vi "johnson.vi"() -> ()   [LabVIEW 2025]
uses:
  <vilib>/Analysis/1siggen.llb/Ramp Pattern by Samples.vi
  <vilib>/Analysis/NI_AALBase.lvlib
panel:
  out "Variance":dbl
  out "Stdev":dbl
  out "Mean":dbl
  out "Waveform Graph":dbl[][](graph)
  out "Output":string
  out "XY Graph":cluster{"Y":dbl[], "Y":dbl[]}[](graph)
  in  "samples":dbl
  in  "V/div":dbl
  in  "s/div":dbl
  in  "VISA resource name":refnum<visa-resource-name>
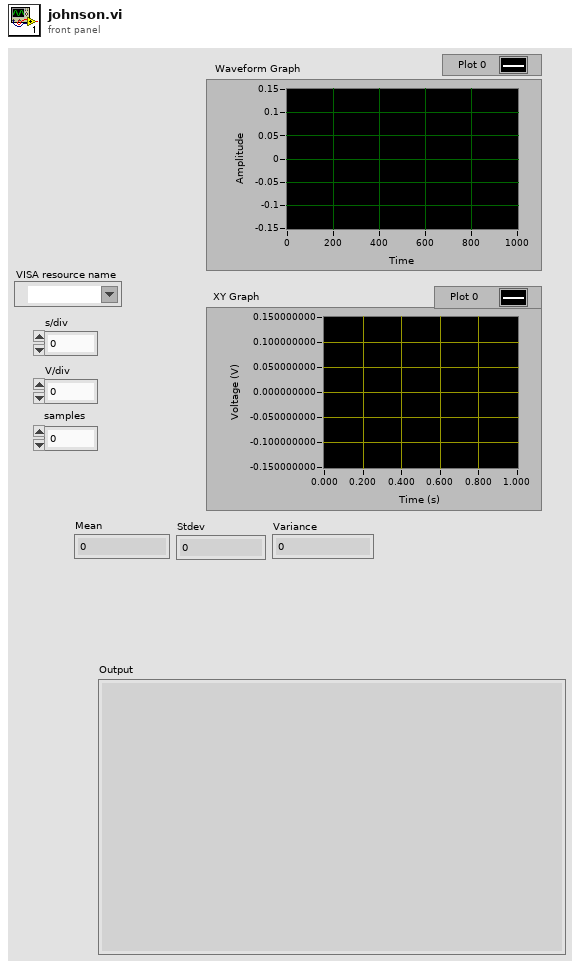
[diagram p1: front panel]
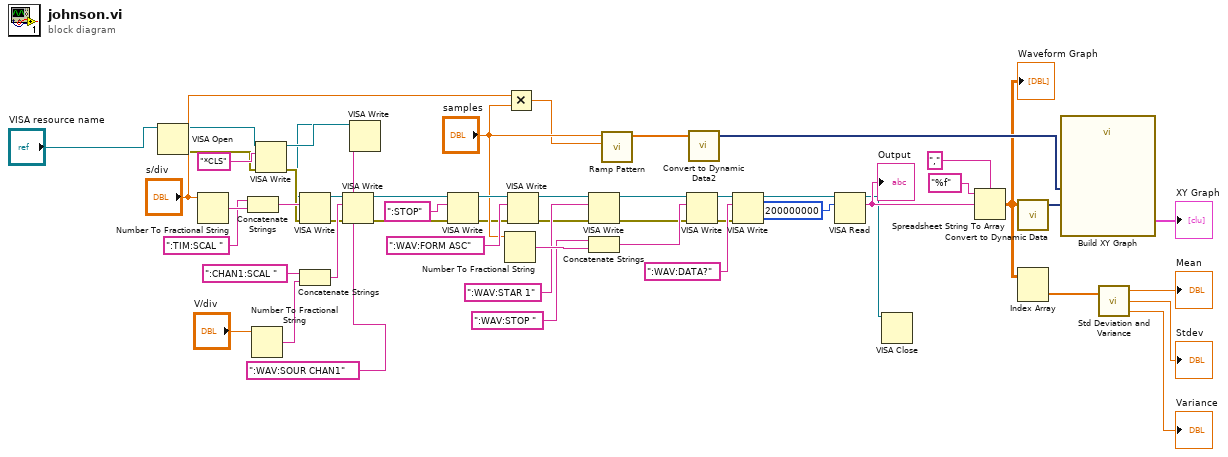
[diagram p0: block diagram]
diagram:
  n1 = VISA Open(VISA resource name="VISA resource name") -> (VISA resource name=w14:refnum<visa-resource-name>, error out=w11:errorcluster)  [unwired: 4 in]
  n2 = Number To Fractional String(number="s/div") -> (F-format string=w52:string)  [unwired: 3 in]
  n3 = Concatenate Strings(":TIM:SCAL ", w52) -> (w50:string)
  n4 = Number To Fractional String(number="V/div") -> (F-format string=w48:string)  [unwired: 3 in]
  n5 = VISA Write(VISA resource name=w14, write buffer="*CLS", error in (no error)=w11) -> (VISA resource name out=w2:refnum<visa-resource-name>, error out=w10:errorcluster)  [unwired: 1 out]
  n6 = Concatenate Strings(":CHAN1:SCAL ", w48) -> (w45:string)
  n7 = VISA Write(VISA resource name=w2, write buffer=":WAV:SOUR CHAN1") -> (VISA resource name out=w1:refnum<visa-resource-name>)  [unwired: 1 in, 2 out]
  n8 = VISA Write(VISA resource name=w1, write buffer=w50, error in (no error)=w10) -> (VISA resource name out=w46:refnum<visa-resource-name>, error out=w9:errorcluster)  [unwired: 1 out]
  n9 = VISA Write(VISA resource name=w46, write buffer=w45, error in (no error)=w9) -> (VISA resource name out=w43:refnum<visa-resource-name>, error out=w8:errorcluster)  [unwired: 1 out]
  n10 = VISA Write(VISA resource name=w43, write buffer=":STOP", error in (no error)=w8) -> (VISA resource name out=w33:refnum<visa-resource-name>, error out=w7:errorcluster)  [unwired: 1 out]
  n11 = Number To Fractional String(number="samples") -> (F-format string=w42:string)  [unwired: 3 in]
  n12 = Multiply(x="s/div", y="samples") -> (x*y=w21:dbl)
  n13 = VISA Write(VISA resource name=w33, write buffer=":WAV:FORM ASC", error in (no error)=w7) -> (VISA resource name out=w31:refnum<visa-resource-name>, error out=w6:errorcluster)  [unwired: 1 out]
  n14 = VISA Write(VISA resource name=w31, write buffer=":WAV:STAR 1", error in (no error)=w6) -> (VISA resource name out=w34:refnum<visa-resource-name>, error out=w5:errorcluster)  [unwired: 1 out]
  n15 = Concatenate Strings(":WAV:STOP ", w42) -> (w40:string)
  n16 = call-poly <vilib>:"Ramp Pattern.vi"("end"=w21, "samples"="samples") -> ("Ramp Pattern"=w28:dbl[])  [unwired: 8 in, 1 out]
  n17 = VISA Write(VISA resource name=w34, write buffer=w40, error in (no error)=w5) -> (VISA resource name out=w38:refnum<visa-resource-name>, error out=w4:errorcluster)  [unwired: 1 out]
  n18 = call "Convert to Dynamic Data2"("Array"=w28) -> ("Dynamic Data Type"=w26:dynamicdata)  [unwired: 3 in]
  n19 = VISA Write(VISA resource name=w38, write buffer=":WAV:DATA?", error in (no error)=w4) -> (VISA resource name out=w37:refnum<visa-resource-name>)  [unwired: 2 out]
  n20 = VISA Read(VISA resource name=w37, byte count=u32 200000000) -> (VISA resource name out=w12:refnum<visa-resource-name>, read buffer=w27:string)  [unwired: 1 in, 2 out]
  "Output" <- w27
  n21 = VISA Close(VISA resource name=w12) -> ()  [unwired: 1 in, 1 out]
  n22 = Spreadsheet String To Array(delimiter (Tab)=",", format string="%f", spreadsheet string=w27) -> (array=w20:dbl[][])  [unwired: 1 in]
  "Waveform Graph" <- w20
  n23 = call "Convert to Dynamic Data"("2D Array"=w20) -> ("Dynamic Data Type"=w30:dynamicdata)  [unwired: 3 in]
  n24 = Index Array(array=w20) -> (element=w19:dbl[])  [unwired: 2 in]
  n25 = call "Build XY Graph"("Y Input"=w30, "X Input"=w26) -> ("XY Graph"=→"XY Graph":cluster{"X":dbl[], "Y":dbl[]}[])  [unwired: 8 in, 1 out]
  n26 = call <vilib>:"Std Deviation and Variance.vi"("X"=w19) -> ("mean"=→"Mean":dbl, "standard deviation"=→"Stdev":dbl, "variance"=→"Variance":dbl)  [unwired: 1 in]
